vi "mxwScript_API_Option_RemoveStructInCleanup.vi"(5 "time":i32, 6 "frameIndex":u32, 7 "structureName":string, 8 "error in (no error)":errorcluster, 9 "templateIndex":i32, 10 "isTerminalID?":bool, 11 "options in":T1[](array[typedef])) -> (0 "error out":errorcluster, 3 "options out":T1[](array[typedef]))   [LabVIEW 2020]
uses:
  codeGenAPISupport.llb/cgAPI_mxwScript_OptionData.ctl
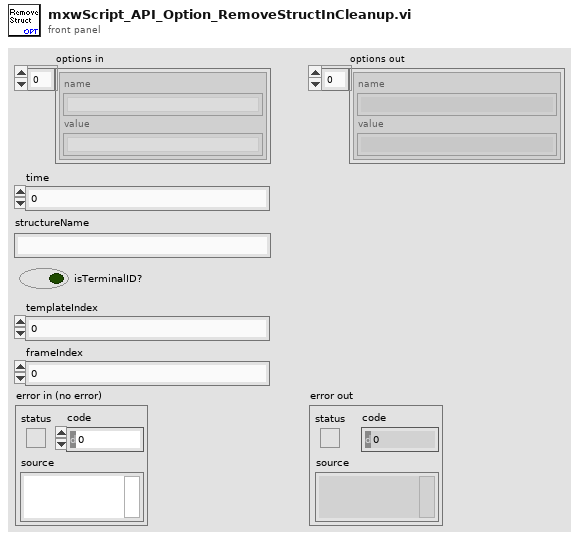
[diagram p1: front panel]
types:
  T1 = typedef "cgAPI_mxwScript_OptionData.ctl" = cluster{"name":string, "value":string}
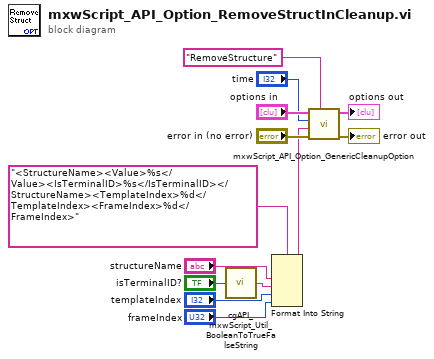
[diagram p0: block diagram]
diagram:
  n1 = call "cgAPI_mxwScript_Util_BooleanToTrueFalseString.vi"("boolean"="isTerminalID?") -> ("TRUE/FALSE text"=w3:string)  [unwired: 4 out]
  n2 = Format Into String(format string="<StructureName><Value>%s</Value><IsTerminalID>%s</IsTerminalID></StructureName><TemplateIndex>%d</TemplateIndex><FrameIndex>%d</FrameIndex>", "structureName", w3, "templateIndex", "frameIndex") -> (resulting string=w5:string)  [unwired: 2 in, 1 out]
  n3 = call "mxwScript_API_Option_GenericCleanupOption.vi"("cleanupOption"="RemoveStructure", "error in (no error)"="error in (no error)", "data"=w5, "time"="time", "options in"="options in") -> ("error out"=→"error out":errorcluster, "options out"=→"options out":T1[])  [unwired: 5 out]
